vi "IND560 Serial Get Data.vi"(8 "error in (no error)":errorcluster, 11 "VISA Refnum in":refnum<visa-resource-name>) -> (0 "error out":errorcluster, 1 "Gross Weight":dbl, 2 "IND560 Serial Data":string[][](array[string]), 3 "VISA Refnum out":refnum<visa-resource-name>)   [LabVIEW 2019]
uses:
  Type Definitions/IND560 Serial Scale Commands.ctl
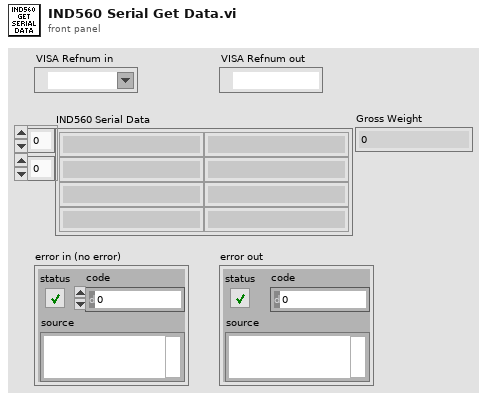
[diagram p1: front panel]
types:
  T1 = typedef "IND560 Serial Scale Commands.ctl" = string
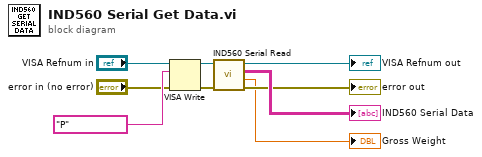
[diagram p0: block diagram]
diagram:
  n1 = VISA Write(VISA resource name="VISA Refnum in", write buffer=T1 "P" ("Scale Commands"), error in (no error)="error in (no error)") -> (VISA resource name out=w5:refnum<visa-resource-name>, error out=w7:errorcluster)  [unwired: 1 out]
  n2 = call "IND560 Serial Read.vi"("error in (no error)"=w7, "VISA Refnum in"=w5) -> ("error out"=→"error out":errorcluster, "Net Weight"=→"Gross Weight":dbl, "IND560 Serial Data"=→"IND560 Serial Data":string[][], "VISA Refnum out"=→"VISA Refnum out":refnum<visa-resource-name>)  [unwired: 6 in]
